vi "principal.vi"() -> ()   [LabVIEW 2024]
uses:
  Control/Menu-States-CTRL.ctl
  <vilib>/Utility/error.llb/DialogType.ctl
panel:
  in  "Enum":T1
  out "Access granted":bool
  in  "Exit":bool
  in  "Menu":T2
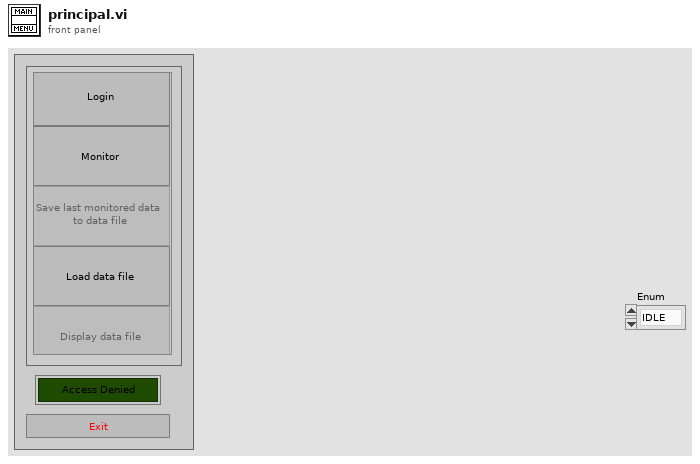
[diagram p1: front panel]
types:
  T1 = typedef "Menu-States-CTRL.ctl" = enum16{"IDLE", "Login", "Monitor", "Save Last", "Load", "Display", "Exit", "Init"}
  T2 = cluster{"Login":bool, "Monitor":bool, "Save Last":bool, "Load data":bool, "Display file":bool}
  T3 = typedef "DialogType.ctl" = u16
  T4 = enum8{"Enabled", "Disabled", "Disabled and Grayed Out"}
  T5 = cluster{"User Name":string, "Time Stamp":timestamp, cluster{"RTD Temp":dbl, "Temp. Max":dbl, "Temp. min":dbl}[]}
  T6 = enum16{"open", "replace", "create", "open or create", "replace or create", "replace or create with confirmation"}
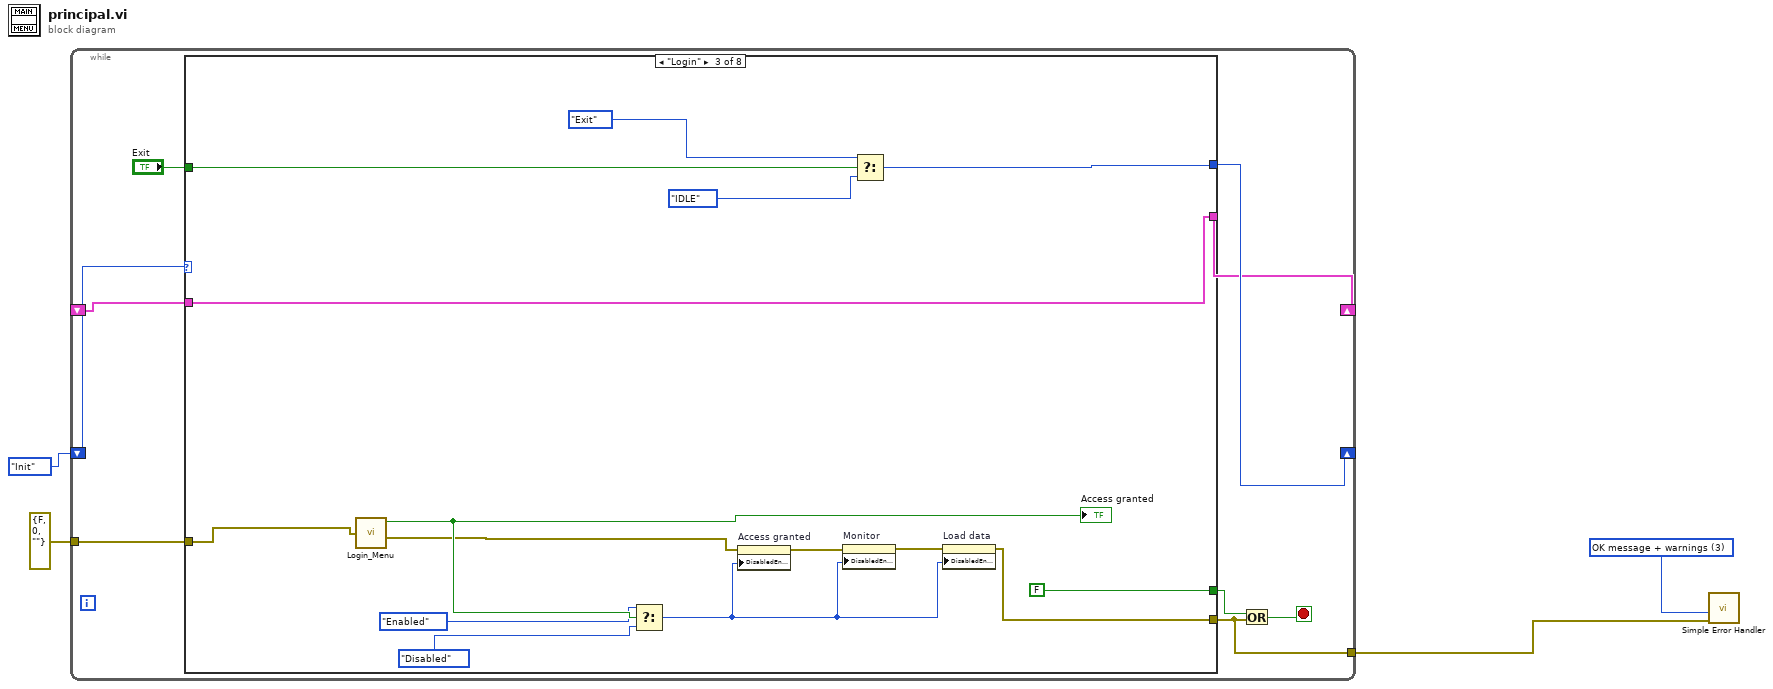
[diagram p0: block diagram]
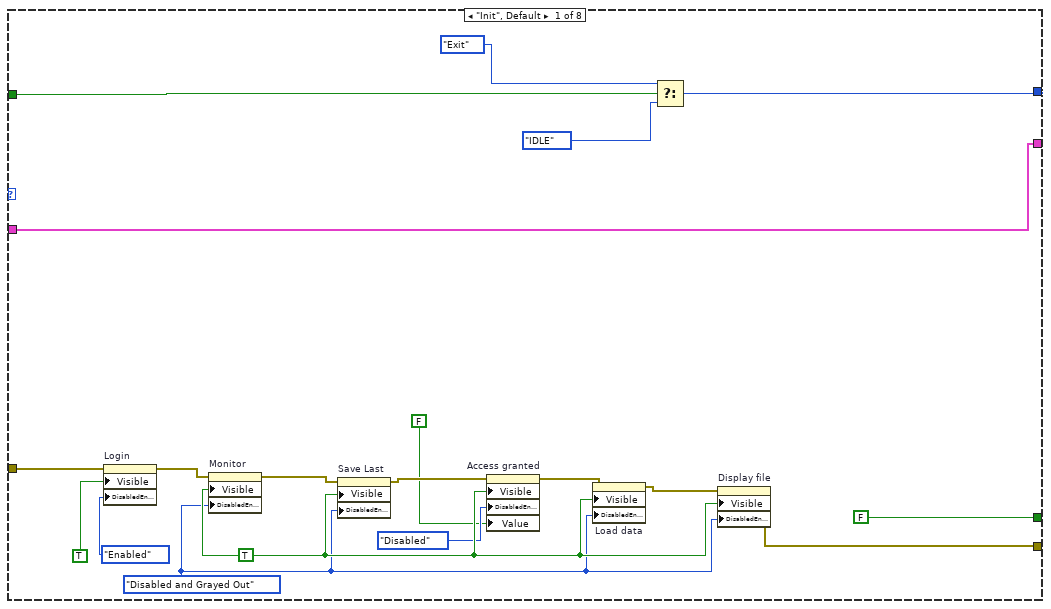
[diagram p2: hidden frame]
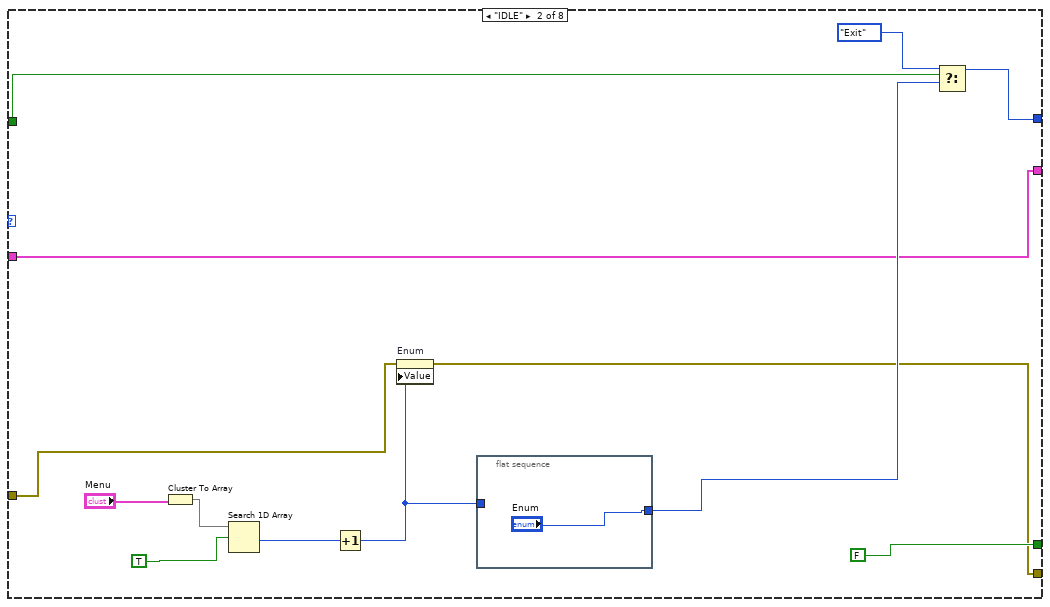
[diagram p3: hidden frame]
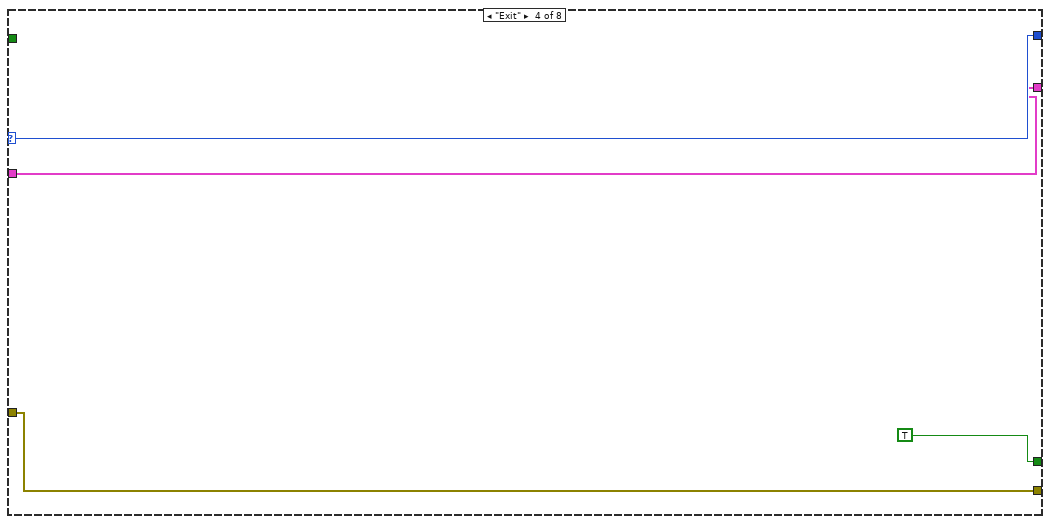
[diagram p4: hidden frame]
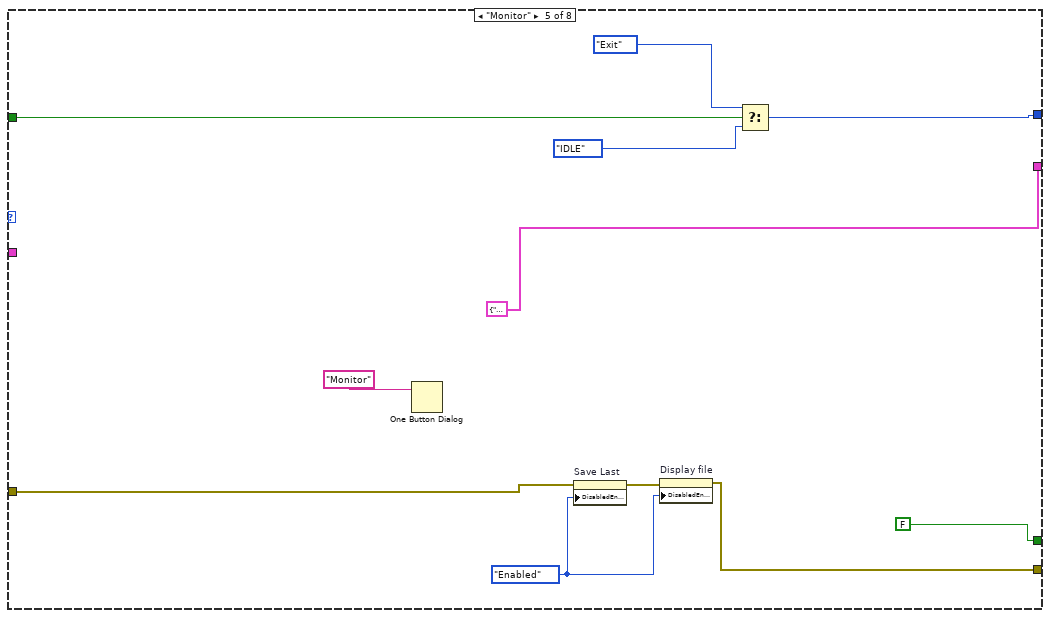
[diagram p5: hidden frame]
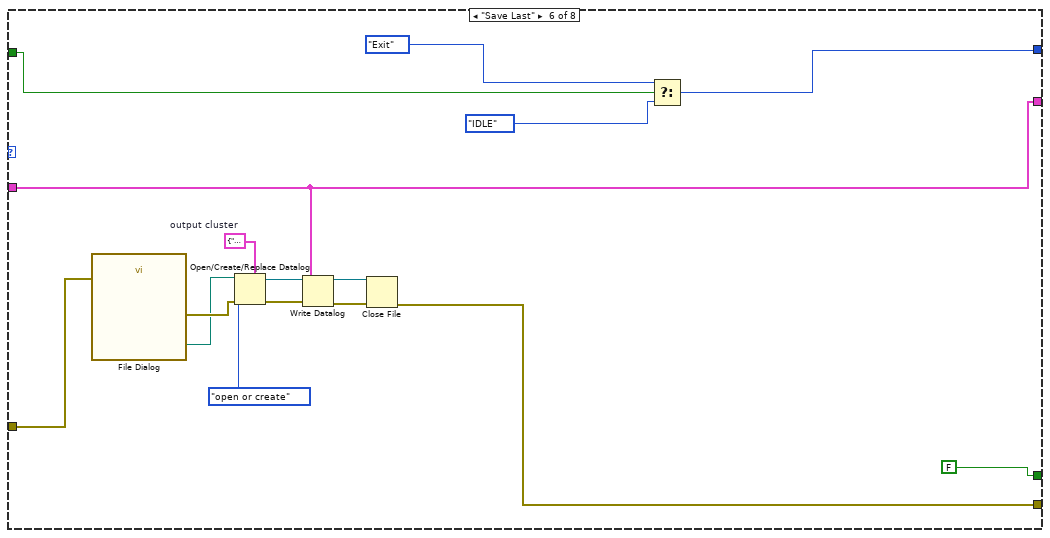
[diagram p6: hidden frame]
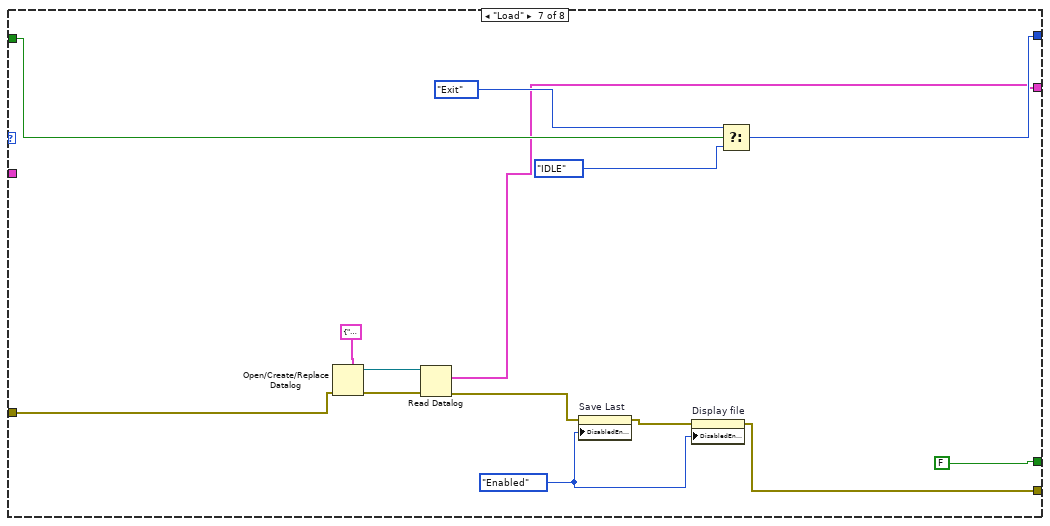
[diagram p7: hidden frame]
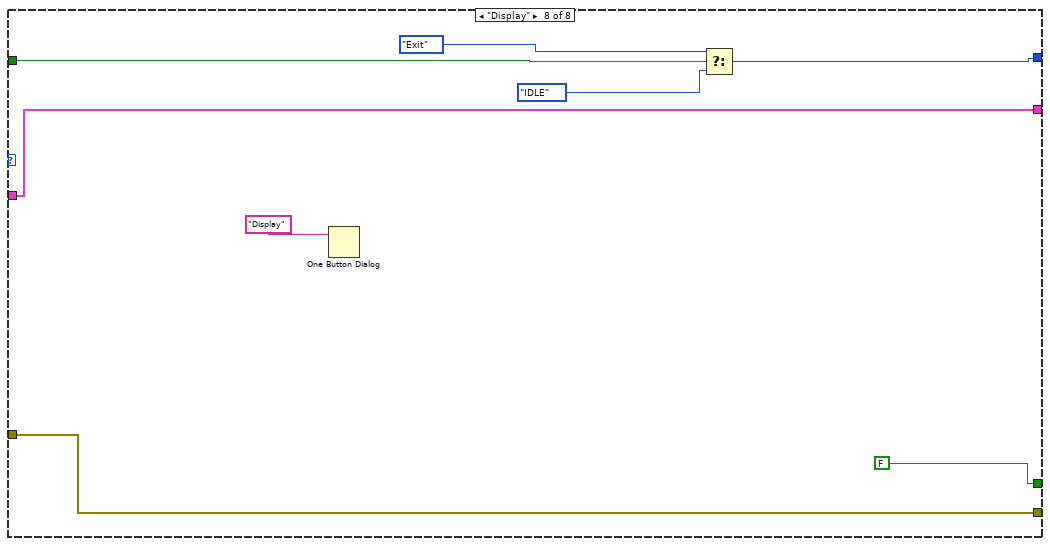
[diagram p8: hidden frame]
diagram:
  w1 = T3 3 items=["no dialog", "OK message", "continue or stop message", "OK message + warnings", "continue/stop + warnings"] ("type of dialog (OK msg:1)")
  n1 = while {
    tunnel: errorcluster {"status"=FALSE, "code"=0, "source"=""} ("error out") -> [w12]
    shift-right: [w11] -> _
    shift-left: Menu-States-CTRL."Init" -> [w13]
    tunnel: [w5] -> w2
    shift-right: [w9] -> _
    shift-left: _ -> [w8]
    stop <- w6 stop-if-true
    n2 = case shown="\"Login\"" w13 {
      selector: w13 -> [_ _ _ w64 _ _ _ _]
      tunnel: w12 -> [w30 w37 w56 w63 w69 w79 w98 w112]
      tunnel: [w24 w36 w48 w63 w67 w78 w94 w112] -> w5
      tunnel: [w19 w41 w59 w64 w72 w89 w102 w109] -> w11
      tunnel: [FALSE FALSE FALSE TRUE FALSE FALSE FALSE FALSE] -> w7
      tunnel: "Exit" -> [w17 w40 w58 _ w71 w88 w103 w108]
      tunnel: w8 -> [w14 w33 w47 w62 _ w77 _ w107]
      tunnel: [w14 w33 w47 w62 T5 {"User Name"="", "Time Stamp"=timestamp(0 s since 1904-01-01), []} ("output cluster") w77 w97 w107] -> w9
      frame "Init", Default {
        w22 = T4."Disabled and Grayed Out" ("Disabled")
        w23 = TRUE ("Visible")
        n3 = property on="Login" class="Bool"(error in=w30, "Visible"=TRUE, "DisabledEnum"=T4."Enabled" ("Disabled")) -> (error out=w29:errorcluster)  [unwired: 1 in, 1 out]
        n4 = property on="Monitor" class="Bool"(error in=w29, "Visible"=w23, "DisabledEnum"=w22) -> (error out=w28:errorcluster)  [unwired: 1 in, 1 out]
        n5 = property on="Save Last" class="Bool"(error in=w28, "Visible"=w23, "DisabledEnum"=w22) -> (error out=w27:errorcluster)  [unwired: 1 in, 1 out]
        n6 = property on="Access granted" class="Bool (strict)"(error in=w27, "Visible"=w23, "DisabledEnum"=T4."Disabled" ("Disabled"), "Value"=FALSE ("Access granted")) -> (error out=w26:errorcluster)  [unwired: 1 in, 1 out]
        n7 = property on="Load data" class="Bool"(error in=w26, "Visible"=w23, "DisabledEnum"=w22) -> (error out=w25:errorcluster)  [unwired: 1 in, 1 out]
        n8 = Select(t=Menu-States-CTRL."Exit" ("Enum"), s=w17, f=Menu-States-CTRL."IDLE") -> (s? t:f=w19:T1)
        n9 = property on="Display file" class="Bool"(error in=w25, "Visible"=w23, "DisabledEnum"=w22) -> (error out=w24:errorcluster)  [unwired: 1 in, 1 out]
      }
      frame "IDLE" {
        n10 = Cluster To Array(cluster="Menu") -> (array=w45:bool[])
        n11 = Search 1D Array(1D array=w45, element=TRUE) -> (index of element=w34:i32)  [unwired: 1 in]
        n12 = Increment(x=w34) -> (x+1=w35:i32)
        n13 = property on="Enum" class="Enum (strict)"(error in=w37, "Value"=w35) -> (error out=w36:errorcluster)  [unwired: 1 in, 1 out]
        n14 = flat-sequence {
          tunnel: ["Enum"] -> w38
          tunnel: w35 -> [_]
          frame #0 {
          }
        }
        n15 = Select(t=Menu-States-CTRL."Exit" ("f"), s=w40, f=w38) -> (s? t:f=w41:T1)
      }
      frame "Login" {
        n16 = call "Login_Menu.vi"("error in (no error)"=w56) -> ("error out"=w51:errorcluster, "Boolean"=w54:bool)  [unwired: 3 in]
        "Access granted" <- w54
        n17 = Select(t=T4."Enabled" ("Disabled"), s=w54, f=T4."Disabled") -> (s? t:f=w52:T4)
        n18 = property on="Access granted" class="Bool (strict)"(error in=w51, "DisabledEnum"=w52) -> (error out=w50:errorcluster)  [unwired: 1 in, 1 out]
        n19 = property on="Monitor" class="Bool"(error in=w50, "DisabledEnum"=w52) -> (error out=w49:errorcluster)  [unwired: 1 in, 1 out]
        n20 = Select(t=Menu-States-CTRL."Exit" ("f"), s=w58, f=Menu-States-CTRL."IDLE") -> (s? t:f=w59:T1)
        n21 = property on="Load data" class="Bool"(error in=w49, "DisabledEnum"=w52) -> (error out=w48:errorcluster)  [unwired: 1 in, 1 out]
      }
      frame "Exit" {
      }
      frame "Monitor" {
        w66 = T4."Enabled" ("Disabled")
        n22 = One Button Dialog(message="Monitor") -> ()  [unwired: 1 in, 1 out]
        n23 = property on="Save Last" class="Bool"(error in=w69, "DisabledEnum"=w66) -> (error out=w68:errorcluster)  [unwired: 1 in, 1 out]
        n24 = property on="Display file" class="Bool"(error in=w68, "DisabledEnum"=w66) -> (error out=w67:errorcluster)  [unwired: 1 in, 1 out]
        n25 = Select(t=Menu-States-CTRL."Exit" ("f"), s=w71, f=Menu-States-CTRL."IDLE") -> (s? t:f=w72:T1)
      }
      frame "Save Last" {
        w84 = T5 {"User Name"="", "Time Stamp"=timestamp(0 s since 1904-01-01), []}  # output cluster
        n26 = call "File Dialog"("error in"=w79) -> ("selected path"=w81:path, "error out"=w87:errorcluster)  [unwired: 11 in, 2 out]
        n27 = Open/Create/Replace Datalog(5:w84, 8:w87, 10:T6."open or create" ("operation (0:open)"), 11:w81) -> (0:w86:errorcluster, 3:w83:refnum<k1>)  [unwired: 2 in, 1 out]
        n28 = Write Datalog(4:w86, 6:w77, 7:w83) -> (0:w85:errorcluster, 3:w82:refnum<k1>)
        n29 = Close File(refnum=w82, error in=w85) -> (error out=w78:errorcluster)  [unwired: 1 out]
        n30 = Select(t=Menu-States-CTRL."Exit" ("f"), s=w88, f=Menu-States-CTRL."IDLE") -> (s? t:f=w89:T1)
      }
      frame "Load" {
        w93 = T4."Enabled" ("Disabled")
        n31 = Open/Create/Replace Datalog(5:T5 {"User Name"="", "Time Stamp"=timestamp(0 s since 1904-01-01), []} ("Historic data"), 8:w98) -> (0:w100:errorcluster, 3:w101:refnum<k1>)  [unwired: 4 in, 1 out]
        n32 = Read Datalog(4:w100, 7:w101) -> (0:w96:errorcluster, 2:w97:T5)  [unwired: 1 in, 1 out]
        n33 = property on="Save Last" class="Bool"(error in=w96, "DisabledEnum"=w93) -> (error out=w95:errorcluster)  [unwired: 1 in, 1 out]
        n34 = property on="Display file" class="Bool"(error in=w95, "DisabledEnum"=w93) -> (error out=w94:errorcluster)  [unwired: 1 in, 1 out]
        n35 = Select(t=Menu-States-CTRL."Exit" ("f"), s=w103, f=Menu-States-CTRL."IDLE") -> (s? t:f=w102:T1)
      }
      frame "Display" {
        n36 = One Button Dialog(message="Display") -> ()  [unwired: 1 in, 1 out]
        n37 = Select(t=Menu-States-CTRL."Exit" ("f"), s=w108, f=Menu-States-CTRL."IDLE") -> (s? t:f=w109:T1)
      }
    }
    n38 = Or(x=w7, y=w5) -> (x .or. y?=w6:bool)
  }
  n39 = call <vilib>:"Simple Error Handler.vi"("type of dialog (OK msg:1)"=w1, "error in (no error)"=w2) -> ()  [unwired: 3 in, 5 out]
